vi "MoveCarriageToPositionAndHold.vi"(6 "Lift Speed":dbl, 7 "Target Height":dbl) -> ()   [LabVIEW 2017]
uses:
  Robot Global Data.vi
  <vilib>/Rock Robotics/WPI/ThirdParty/Phoenix-LabVIEW/Motor Controller/Get/CTRE_Phoenix_MotorController_GetLimitSwitchStates.vi
  <vilib>/Rock Robotics/Network Tables/NT Write Number.vi
  <vilib>/addons/control/pid/pid.llb/PID (DBL).vi
  <vilib>/addons/control/pid/NI_PID_pid.lvlib
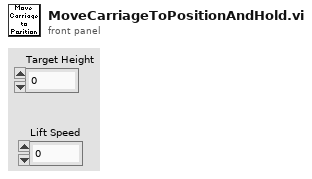
[diagram p1: front panel]
types:
  T1 = typedef "WPI_MotorControlDeviceRef.ctl" = cluster{"DeviceStatus":errorcluster, "Type":T2, "PWM":cluster{"PWM Channel":T3, "DeadBand":T4}, "CAN":cluster{"Device Number":u8, "SetOutput VI Ref":variant, "GetOutput VI Ref":variant, "Enable VI Ref":variant, "Disable VI Ref":variant, "Data":variant}, "Invert":bool, "DIO PWM":cluster{"PWM \"Enable\" Channel":T3, "DIOChannel":T5, "PWM Rate":dbl}}
  T2 = typedef "WPI_MotorControlType.ctl" = enum16{"PWM", "CAN", "DIO PWM"}
  T3 = typedef "FPGA_DIOPWMChannel.ctl" = enum8{"PWM 0", "PWM 1", "PWM 2", "PWM 3", "PWM 4", "PWM 5", "PWM 6", "PWM 7", "PWM 8", "PWM 9", "PWM MXP 0", "PWM MXP 1", "PWM MXP 2", "PWM MXP 3", "PWM MXP 4", "PWM MXP 5", "PWM MXP 6", "PWM MXP 7", "PWM MXP 8", "PWM MXP 9", "Invalid"}
  T4 = typedef "WPI_PWMDeadband.ctl" = cluster{"Name":string, "maxPositivePwm":i32, "minPositivePwm":i32, "centerPwm":i32, "maxNegativePwm":i32, "minNegativePwm":i32, "angularRange":u16}
  T5 = typedef "FPGA_DIOChannel.ctl" = enum8{"DIO 0", "DIO 1", "DIO 2", "DIO 3", "DIO 4", "DIO 5", "DIO 6", "DIO 7", "DIO 8", "DIO 9", "DIO MXP 0", "DIO MXP 1", "DIO MXP 2", "DIO MXP 3", "DIO MXP 4", "DIO MXP 5", "DIO MXP 6", "DIO MXP 7", "DIO MXP 8", "DIO MXP 9", "DIO MXP 10", "DIO MXP 11", "DIO MXP 12", "DIO MXP 13", "DIO MXP 14", "DIO MXP 15", "SPI Port CS1", "SPI Port CS2", "SPI Port CS3", "SPI Port MISO", "SPI Port MOSI", "Invalid"}
  T6 = cluster{"proportional gain (Kc)":dbl, "integral time (Ti, min)":dbl, "derivative time (Td, min)":dbl}
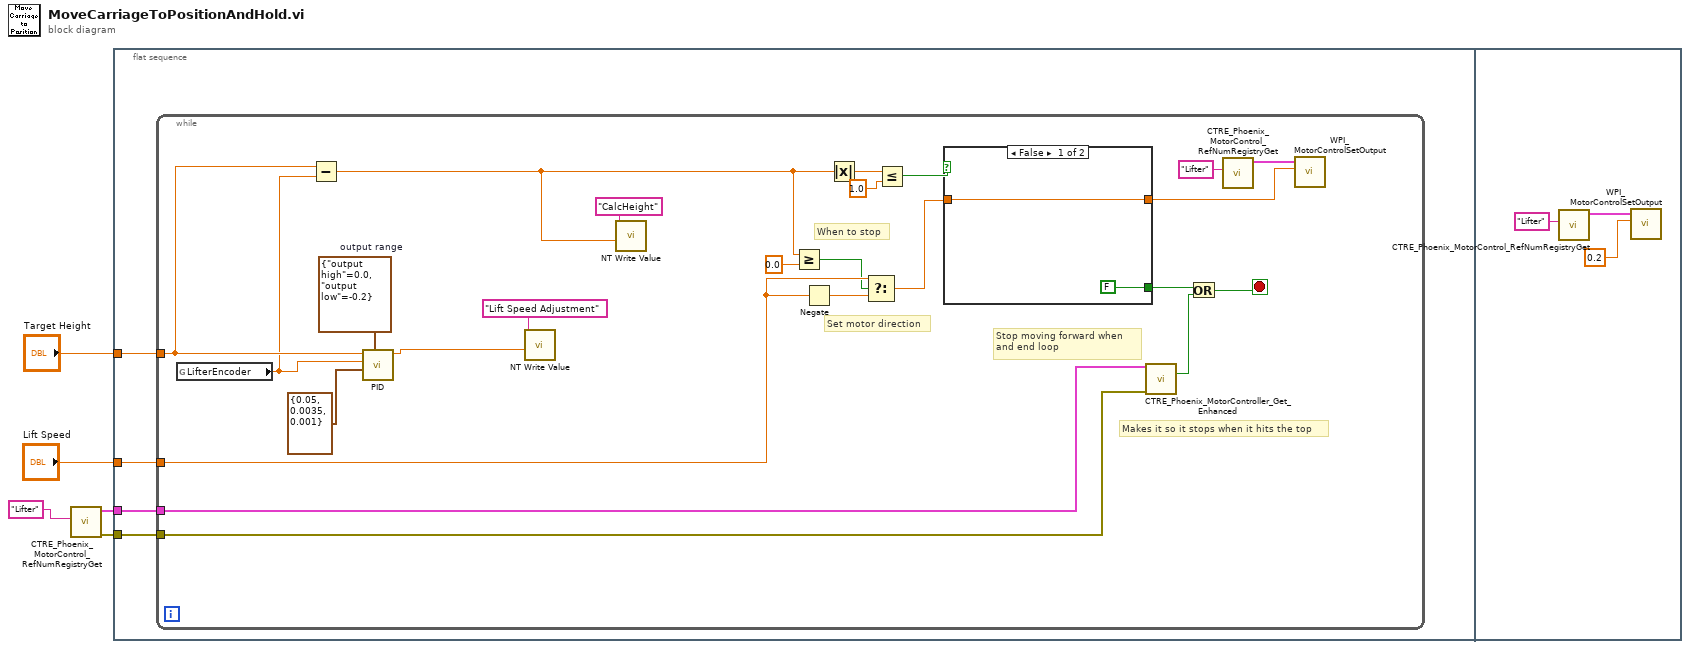
[diagram p0: block diagram]
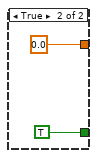
[diagram p2: hidden frame]
diagram:
  n1 = call <vilib>:"CTRE_Phoenix_MotorControl_RefNumRegistryGet.vi"("refnum name"="Lifter") -> ("error out"=w2:errorcluster, "PhoenixMotorControlDevRef"=w1:T1)  [unwired: 9 in]
  n2 = flat-sequence {
    tunnel: "Target Height" -> [w8]
    tunnel: "Lift Speed" -> [w9]
    tunnel: w2 -> [w7]
    tunnel: w1 -> [w6]
    frame #0 {
      n3 = while {
        tunnel: w9 -> [w23]
        tunnel: w8 -> [w31]
        tunnel: w7 -> [w14]
        tunnel: w6 -> [w10]
        stop <- w13 stop-if-true
        w32 = cluster{"output high":dbl, "output low":dbl} {"output high"=0.0, "output low"=-0.2}  # output range
        # "Makes it so it stops when it hits the top"
        # "Set motor direction"
        # "When to stop"
        # "Stop moving forward when\nand end loop"
        n4 = global read "Robot Global Data.vi" "LifterEncoder"() -> (w30:dbl)
        n5 = Subtract(x=w31, y=w30) -> (x-y=w15:dbl)
        n6 = call-poly <vilib>:"PID.vi"("output range"=w32, "PID gains"=T6 {"proportional gain (Kc)"=0.05, "integral time (Ti, min)"=0.0035, "derivative time (Td, min)"=0.001}, "process variable"=w30, "setpoint"=w31) -> ("output"=w20:dbl)  [unwired: 6 in, 1 out]
        n7 = call-poly <vilib>:"NT Write Value.vi"("Numeric"=w20, "Name"="Lift Speed Adjustment") -> ()  [unwired: 9 in, 1 out]
        n8 = call-poly <vilib>:"NT Write Value.vi"("Numeric"=w15, "Name"="CalcHeight") -> ()  [unwired: 9 in, 1 out]
        n9 = Greater Or Equal?(x=w15, y=0.0) -> (x >= y?=w21:bool)
        n10 = Negate(x=w23) -> (-x=w24:dbl)
        n11 = Absolute Value(x=w15) -> (abs(x)=w18:dbl)
        n12 = Select(t=w23, s=w21, f=w24) -> (s? t:f=w25:dbl)
        n13 = Less Or Equal?(x=w18, y=1.0) -> (x <= y?=w29:bool)
        n14 = case shown="False" w29 {
          tunnel: [FALSE TRUE] -> w12
          tunnel: w25 -> [w34 _]
          tunnel: [w34 0.0] -> w26
          frame False {
          }
          frame True {
          }
        }
        n15 = call-poly <vilib>:"CTRE_Phoenix_MotorController_Get_Enhanced.vi"("PhoenixMotorControlDevRef"=w10, "error in"=w14) -> ("Forward Limit Closed?"=w11:bool)  [unwired: 10 in, 3 out]
        n16 = Or(x=w12, y=w11) -> (x .or. y?=w13:bool)
        n17 = call <vilib>:"CTRE_Phoenix_MotorControl_RefNumRegistryGet.vi"("refnum name"="Lifter") -> ("PhoenixMotorControlDevRef"=w27:T1)  [unwired: 9 in, 1 out]
        n18 = call <vilib>:"WPI_MotorControlSetOutput.vi"("Output"=w26, "MotorControlDevRef"=w27) -> ()  [unwired: 7 in, 3 out]
      }
    }
    frame #1 {
      n19 = call <vilib>:"CTRE_Phoenix_MotorControl_RefNumRegistryGet.vi"("refnum name"="Lifter") -> ("PhoenixMotorControlDevRef"=w39:T1)  [unwired: 9 in, 1 out]
      n20 = call <vilib>:"WPI_MotorControlSetOutput.vi"("Output"=0.2, "MotorControlDevRef"=w39) -> ()  [unwired: 7 in, 3 out]
    }
  }
